vi "PAM Parse MFC Sequence File.vi"(8 "error in":errorcluster, 11 "Sequence File":path) -> (0 "error out":errorcluster, 1 "Time (Last)":dbl, 3 "Cluster Out":T1(array[cluster]))   [LabVIEW 2011]
uses:
  <vilib>/regexp/Match Regular Expression.xnode
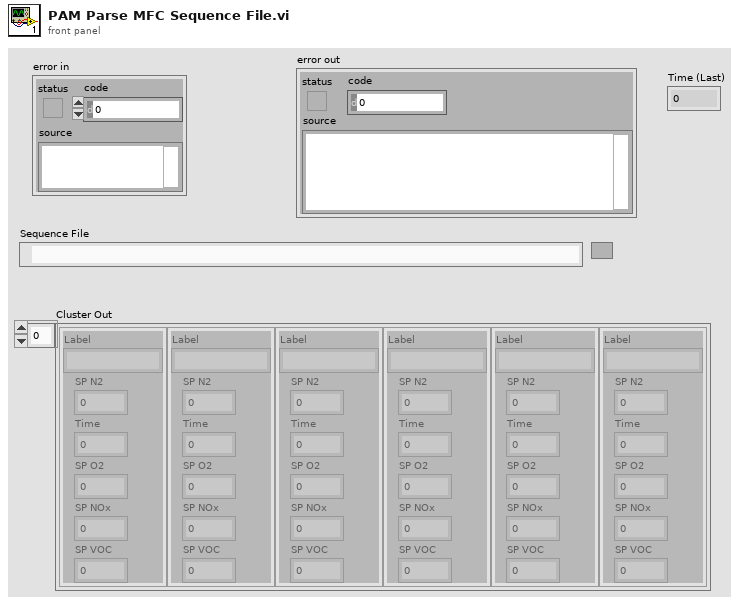
[diagram p1: front panel]
types:
  T1 = cluster{"Label":string, "SP N2":dbl, "Time":dbl, "SP O2":dbl, "SP NOx":dbl, "SP VOC":dbl}[]
  T2 = cluster{"Label":string, "SP N2":dbl, "Time":dbl, "SP O2":dbl, "SP NOx":dbl, "SP VOC":dbl}
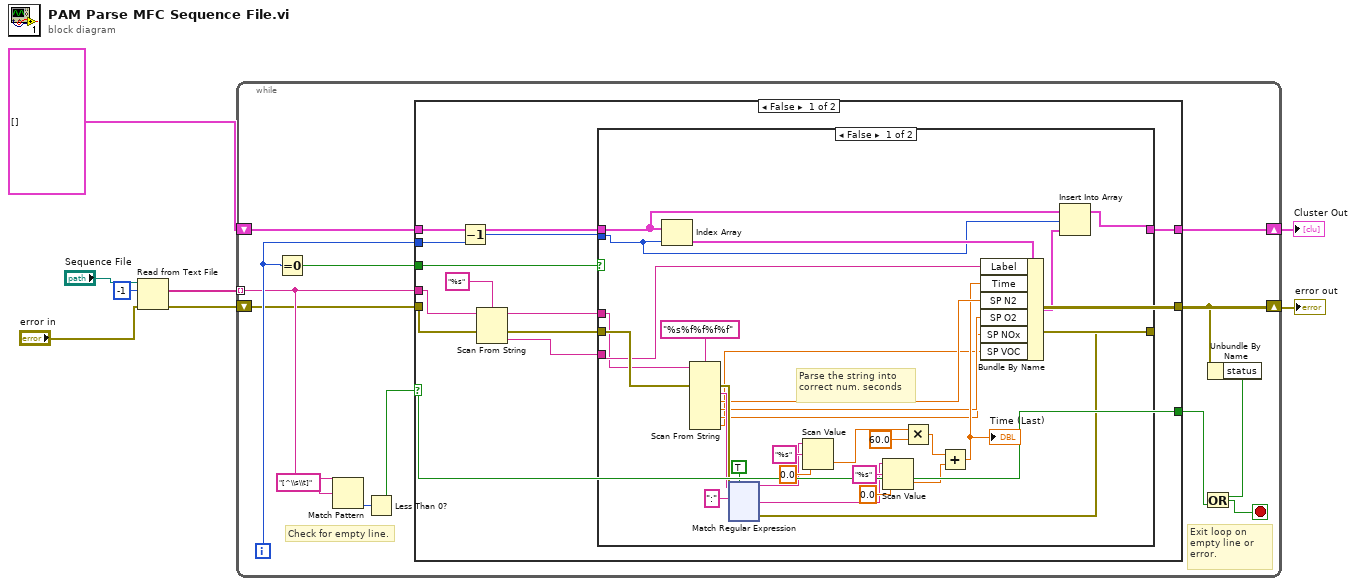
[diagram p0: block diagram]
diagram:
  n1 = Read from Text File(file (use dialog)="Sequence File", count=-1, error in="error in") -> (text=w6:string[], error out=w4:errorcluster)  [unwired: 1 in, 2 out]
  n2 = while {
    tunnel: w6 -> [w15] mode=indexing
    shift-right: [w13] -> w3
    shift-left: w4 -> [w14]
    shift-right: [w10] -> w1
    shift-left: T1 [] -> [w9]
    i -> [w17]
    stop <- w21 stop-if-true
    # "Exit loop on empty line or error."
    # "Check for empty line."
    n3 = Equal To 0?(x=w17) -> (x = 0?=w16:bool)
    n4 = Match Pattern(string=w15, regular expression="[^\\s\\t]") -> (offset past match=w19:i32)  [unwired: 1 in, 3 out]
    n5 = Less Than 0?(x=w19) -> (x < 0?=w18:bool)
    n6 = case shown="False" w18 {
      selector: w18 -> [w22 w178]
      tunnel: w17 -> [w34 _]
      tunnel: w16 -> [w32 _]
      tunnel: w15 -> [w31 _]
      tunnel: w14 -> [w30 w179]
      tunnel: [w23 w179] -> w13
      tunnel: [w22 w178] -> w11
      tunnel: [w25 w177] -> w10
      tunnel: w9 -> [w24 w177]
      frame False {
        n7 = Decrement(x=w34) -> (x-1=w33:i32)
        n8 = Scan From String(format string="%s", input string=w31, error in=w30) -> (remaining string=w28:string, error out=w29:errorcluster, output 1=w26:string)  [unwired: 2 in, 1 out]
        n9 = case shown="False" w32 {
          tunnel: w33 -> [w60 _]
          tunnel: w29 -> [w57 w176]
          tunnel: w28 -> [w55 _]
          tunnel: w26 -> [w56 _]
          tunnel: [w51 w176] -> w23
          tunnel: [w58 w175] -> w25
          tunnel: w24 -> [w59 w175]
          frame False {
            # "Parse the string into correct num. seconds"
            n10 = Index Array(array=w59, index=w60) -> (element=w62:T2)
            n11 = Scan From String(format string="%s%f%f%f%f", input string=w55, error in=w57) -> (error out=w52:errorcluster, output 1=w40:string, output 2=w39:dbl, output 3=w37:dbl, output 4=w36:dbl, output 5=w35:dbl)  [unwired: 6 in, 2 out]
            n12 = xnode "Match Regular Expression"("input string"=w40, "regular expression"=":", "error in"=w52, "ignore case? (F)"=TRUE) -> ("before match"=w48:string, "after match"=w45:string, "error out"=w51:errorcluster)  [unwired: 2 in, 2 out]
            n13 = Scan Value(string=w48, format string="%s", default (0 dbl)=0.0) -> (value=w42:dbl)  [unwired: 1 out]
            n14 = Scan Value(string=w45, format string="%s", default (0 dbl)=0.0) -> (value=w41:dbl)  [unwired: 1 out]
            n15 = Multiply(x=w42, y=60.0) -> (x*y=w43:dbl)
            n16 = Add(x=w43, y=w41) -> (x+y=w38:dbl)
            "Time (Last)" <- w38
            n17 = Bundle By Name(cluster=w62, "Label"=w56, "Time"=w38, "SP N2"=w39, "SP O2"=w37, "SP NOx"=w36, "SP VOC"=w35) -> (w63:T2)
            n18 = Insert Into Array(array=w59, index=w60, new element=w63) -> (w58:T1)
          }
          frame True {
            # "Do nothing - this is the first line of the file, which is a comment."
          }
        }
      }
      frame True {
      }
    }
    n19 = Unbundle By Name(w13) -> ("status"=w12:bool)
    n20 = Or(x=w12, y=w11) -> (x .or. y?=w21:bool)
  }
  "error out" <- w3
  "Cluster Out" <- w1
